vi "PCI-7830R Example.vi"   [LabVIEW 2017]
uses:
  <vilib>/Platform/TimedLoop/XDataNode/timing_clust.ctl
  <vilib>/Platform/TimedLoop/XDataNode/nitl_modes.ctl
  <vilib>/Platform/TimedLoop/XDataNode/wakeup.ctl
  <vilib>/rvi/FXPMathLib/basic elements/FxpIntAccumulator/subVIs/nifxpmath_IntAccumulator_SimConfig.ctl
  <vilib>/rvi/FXPMathLib/FxpSqrt/subVIs/nifxpmath_Sqrt_SimConfig.ctl
  <vilib>/fxp/LVFixedPointOverflowPolicyTypeDef.ctl
  <vilib>/rvi/Emulation/niFpgaSctlEmulationGetInTimedLoop.vi
  <vilib>/rvi/Emulation/niFpgaEmulationReportErrorSimple.vi
  <vilib>/rvi/Emulation/niFpgaGetClockAttributes.vi
  <vilib>/rvi/Emulation/niFpgaCriticalErrorInLSC.vi
  <vilib>/rvi/eio/common/nirviEmuTemplateMethod_errors.vi
  <vilib>/rvi/Analysis/common/codeGenErrors/XNode/niFpgaXNodeCodeGenErrorHandle.vi
  <vilib>/rvi/FXPMathLib/basic elements/FxpIntAccumulator/simVIs/DllFxpIntAccumulator_sub.vi
  <vilib>/rvi/FXPMathLib/FxpSqrt/simVIs/DllSqrtTemp_sub.vi
  <userlib>/_VeriStand FPGA XML Builder/Boolean Array to U64.vi
  <vilib>/NI Veristand/FPGA/NI VeriStand - Send Packet to Host.vi
  <vilib>/Platform/TimedLoop/XDataNode/XDataNode.xnode
  <vilib>/eio/EIONode/EIONode.xnode
  <vilib>/rvi/Analysis/measure/dc-rms/XNode/niFpgaDC-RMS.xnode
  <vilib>/rvi/FXPMathLib/basic elements/FxpIntAccumulator/XNode/nifxpmath_IntAccumulator.xnode
  <vilib>/rvi/FXPMathLib/FxpMul/XNode/nifxpmath_Multiplier.xnode
  <vilib>/rvi/FXPMathLib/FxpSqrt/XNode/nifxpmath_Sqrt.xnode
  <userlib>/_VeriStand FPGA XML Builder/FPGA XML.xnode
  <vilib>/Platform/TimedLoop/XDataNode/XDNodeRunTimeDep.lvlib
  <userlib>/_NI VeriStand FPGA Support/NI VeriStand FPGA Clock Support/NI_VS FPGA Clock Support.lvlib
  <vilib>/rvi/FXPMathLib/sim/FxpSim.dll
  <vilib>/NI Veristand/FPGA/NI_VS FPGA Support.lvlib
panel:
  # "PWM"
  # "Configuration"
types:
  T1 = typedef "XDNodeRunTimeDep.lvlib/timing_clust.ctl" = cluster{"Expected End [f-1]":u64, "Actual End [f-1]":u64, "Finished Late? [f-1]":bool, "Expected End [i-1]":u64, "Actual End [i-1]":u64, "Finished Late? [i-1]":bool, "Expected Start [i]":u64, "Actual Start [i]":u64, "Expected Start [f]":u64, "Actual Start [f]":u64, "Source Name":string, "Structure Name":string, "Period":i64, "Deadline":i64, "Offset":i64, "Start":i64, "Priority":i32, "Timeout":i32, "Mode":T2, "Wakeup Reason":T3, "Error":errorcluster, "Source Type":string, "Secondary Source Type":string, "Global End Time":u64, "Global Start Time":u64, "Frame Duration":u64, "Iteration Duration":u64, "Assigned CPU":i32, "I/O Scan Engine Mode":u32}
  T2 = typedef "XDNodeRunTimeDep.lvlib/nitl_modes.ctl" = enum32{"No Change", "Process missed periods, maintain original phase", "Discard missed periods, maintain original phase", "Process missed periods, ignore original phase", "Discard missed periods, ignore original phase"}
  T3 = typedef "XDNodeRunTimeDep.lvlib/wakeup.ctl" = enum32{"Normal", "Aborted", "Asynchronous wakeup", "Timing source error", "Timed loop error", "Timeout"}
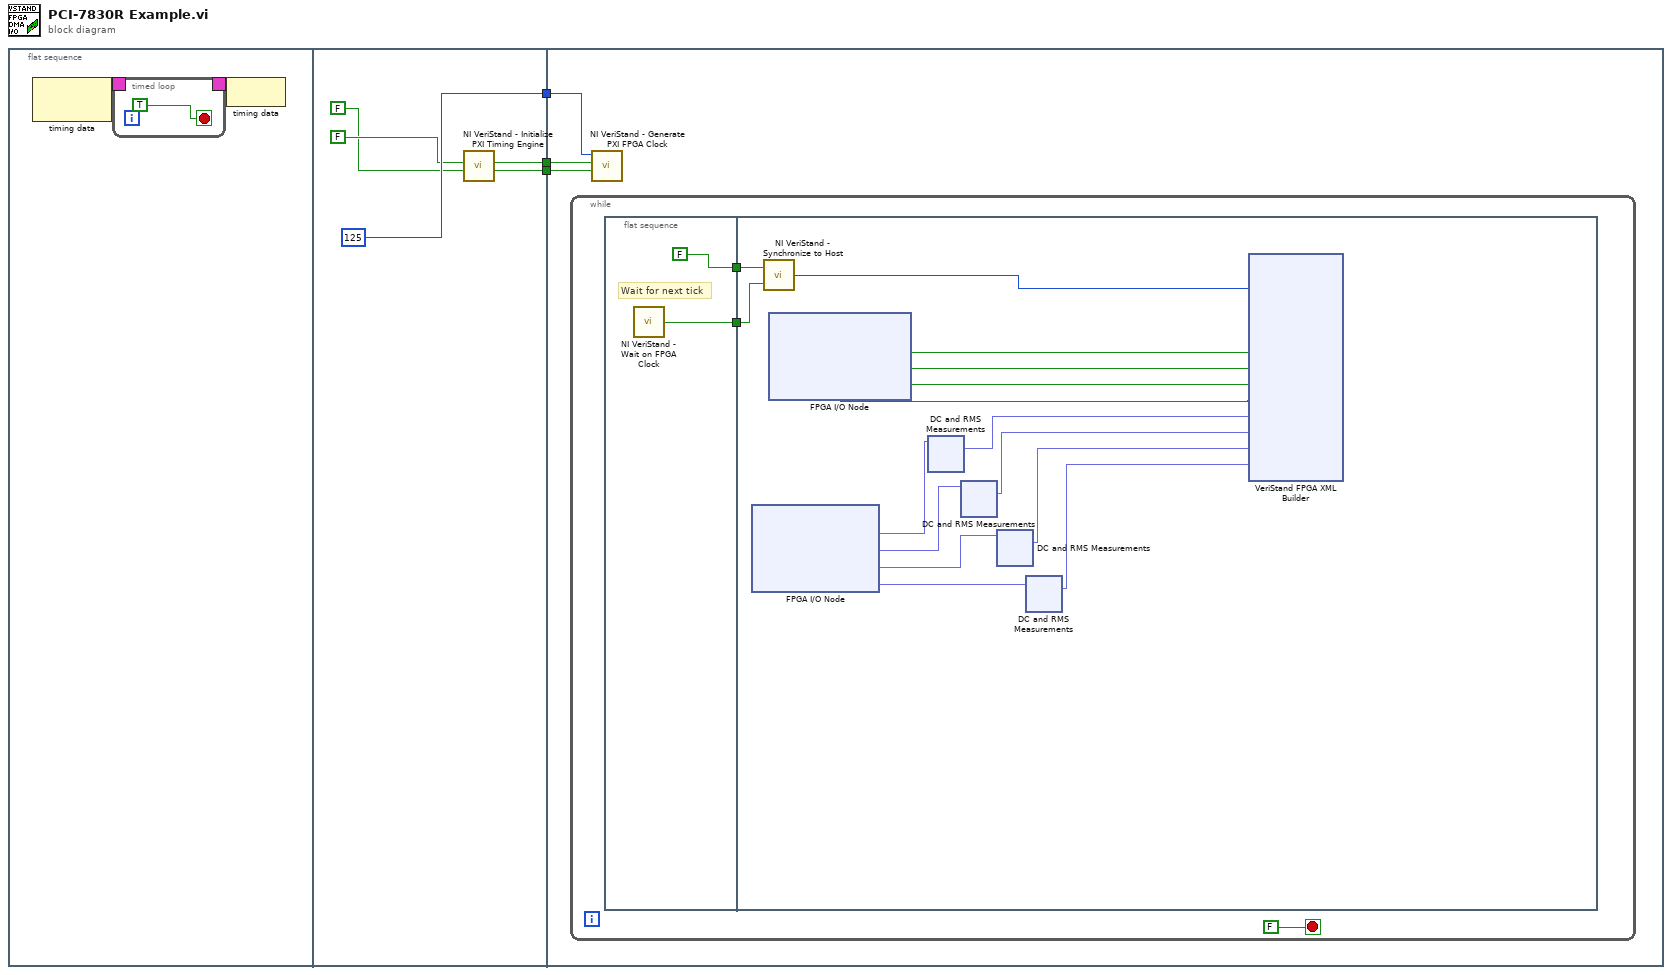
[diagram p0: block diagram]
diagram:
  n1 = flat-sequence {
    tunnel: [w11] -> w3
    tunnel: [u32 125 ("Loop Rate (usec)")] -> w2
    tunnel: [w12] -> w1
    tunnel: w3 -> [w18]
    tunnel: w2 -> [w17]
    tunnel: w1 -> [w16]
    frame #0 {
      n2 = node-c288() -> (w5:T1)  [unwired: 1 out]
      n3 = timed-loop {
        timing: w5 -> [_]
        timing-out: [_] -> w4
        stop <- TRUE ("Start") stop-if-true
      }
      n4 = node-c288(w4) -> ()
    }
    frame #1 {
      n5 = call <userlib>:"NI VeriStand - Initialize PXI Timing Engine.vi"("Use External Timing In"=FALSE ("Use External Timing"), "Write to  RTSI In"=FALSE ("Write to  RTSI")) -> ("Use External Timing Out"=w11:bool, "Write to  RTSI Out"=w12:bool)  [unwired: 8 in]
    }
    frame #2 {
      n6 = while {
        stop <- FALSE stop-if-true
        n7 = flat-sequence {
          tunnel: [FALSE ("Generate IRQ")] -> w20
          tunnel: [w22] -> w19
          tunnel: w20 -> [w38]
          tunnel: w19 -> [w37]
          frame #0 {
            # "Wait for next tick"
            n8 = call <userlib>:"NI VeriStand - Wait on FPGA Clock.vi"() -> ("Clock Ticked"=w22:bool)
          }
          frame #1 {
            n9 = xnode "FPGA I/O Node"() -> ("Connector0/AI0"=w31:fxp<+/-,27,5>, "Connector0/AI1"=w30:fxp<+/-,27,5>, "Connector0/AI2"=w29:fxp<+/-,27,5>, "Connector0/AI3"=w28:fxp<+/-,27,5>)  [unwired: 4 in, 4 out]
            n10 = call <userlib>:"NI VeriStand - Synchronize to Host.vi"("Clock Ticked"=w37, "Generate IRQ"=w38) -> ("Is Late?"=w36:u64)
            n11 = xnode "FPGA I/O Node"() -> ("Connector1/DIO16"=w35:bool, "Connector1/DIO17"=w34:bool, "Connector1/DIO18"=w33:bool, "Connector1/DIO19"=w32:bool)  [unwired: 4 in, 4 out]
            n12 = xnode "DC and RMS Measurements"("input data"=w31) -> ("RMS"=w24:fxp<+,27,5>)  [unwired: 1 in, 1 out]
            n13 = xnode "DC and RMS Measurements"("input data"=w30) -> ("RMS"=w25:fxp<+,27,5>)  [unwired: 1 in, 1 out]
            n14 = xnode "DC and RMS Measurements"("input data"=w29) -> ("RMS"=w26:fxp<+,27,5>)  [unwired: 1 in, 1 out]
            n15 = xnode "DC and RMS Measurements"("input data"=w28) -> ("RMS"=w27:fxp<+,27,5>)  [unwired: 1 in, 1 out]
            n16 = xnode "VeriStand FPGA XML Builder"("Timing"=w36, "Connector1/DIO16"=w35, "Connector1/DIO17"=w34, "Connector1/DIO18"=w33, "Connector1/DIO19"=w32, "RMS1"=w24, "RMS2"=w25, "RMS3"=w26, "RMS4"=w27) -> ()
          }
        }
      }
      n17 = call <userlib>:"NI VeriStand - Generate PXI FPGA Clock.vi"("Use External Timing"=w18, "Write to  RTSI"=w16, "Loop Rate (usec)"=w17) -> ()  [unwired: 9 in]
    }
  }
